vi "NI OCR-Main.vi"() -> ()   [LabVIEW 2016]
panel:
  in  "OCR":bool
  in  "Start Training":bool
  in  "Detect Characters":bool
  in  "Import Picture":bool
  out "Display Image":T1(plugin-control)
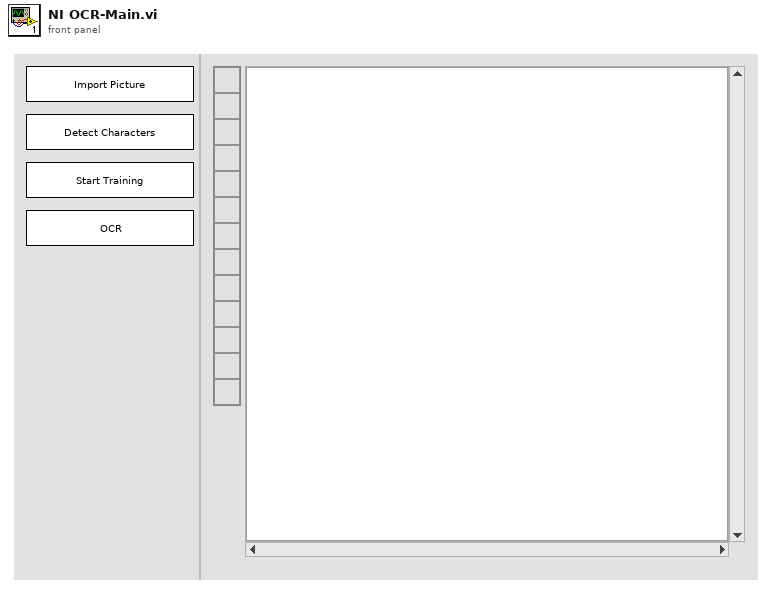
[diagram p1: front panel]
types:
  T1 = typedef "IMAQ Image.ctl" = refnum<image>
  T2 = typedef "NI OCR-Buffer Data.ctl" = cluster{"VI Refnum":refnum<vi>, "Src Image":T1, "Dst Image":T1, "Ctl Refnum []":refnum<vi>[], "Ctl Label":string[], "User Event":refnum<user-event>, "Event Registration Refnum":refnum<event-registration>, "Timeout":i32, "IMAQ OCR Session":T3, "Objects":cluster{"Object Center":cluster{"X":sgl, "Y":sgl}, "Bounding Box":cluster{"X Left":i32, "Y Top":i32, "X Right":i32, "Y Bottom":i32}, "Area":sgl, "Orientation":sgl, "Aspect Ratio":sgl, "Nb Holes":i32}[], "ROI Descriptor":T4, "Settings":cluster{"Objects":u16, "Threshold":i32, "Reject Border":bool, "Fill Holes":bool, "Min Object Size":bool, "Min Size":i32, "Max Object Size":bool, "Max Size":i32, "Show Search Area":bool, "Show Center":bool, "Show Bounding Box":bool}}
  T3 = typedef "IMAQ OCR Session.ctl" = refnum<k1>
  T4 = typedef "ROI Descriptor" = cluster{"Global Rectangle":i32[], "Contours":cluster{"ID":enum32{"External", "Internal"}, "Type":u32, "Coordinates":i32[]}[]}
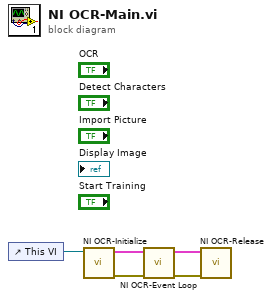
[diagram p0: block diagram]
diagram:
  n1 = control-ref of="This VI"() -> (w5:refnum<vi>)
  n2 = call "NI OCR-Initialize.vi"("VI Refnum"=w5) -> ("error out"=w4:errorcluster, "Buffer Data"=w3:T2)  [unwired: 9 in]
  n3 = call "NI OCR-Event Loop.vi"("error in"=w4, "Buffer Data In"=w3) -> ("error out"=w1:errorcluster, "Buffer Data Out"=w2:T2)  [unwired: 8 in]
  n4 = call "NI OCR-Release.vi"("error in"=w1, "Buffer Data"=w2) -> ()  [unwired: 9 in, 1 out]
